vi "Lab Suma total de los valores de un arreglo.vi"() -> ()   [LabVIEW 2018]
uses:
  <vilib>/Analysis/baseanly.llb/Mean (DBL).vi
  <vilib>/Analysis/NI_AALBase.lvlib
panel:
  out "Numeric 2":dbl
  out "promedio":dbl format="%0.2f"
  out "Minimo Indexado":i32
  out "Maximo Indexado":i32
  out "Minimo":dbl
  out "Maximo":dbl
  out "Array":dbl[](array[numeric])
  out "Numeric":dbl
  in  "Knob":dbl(knob) scale=0.0..10.0
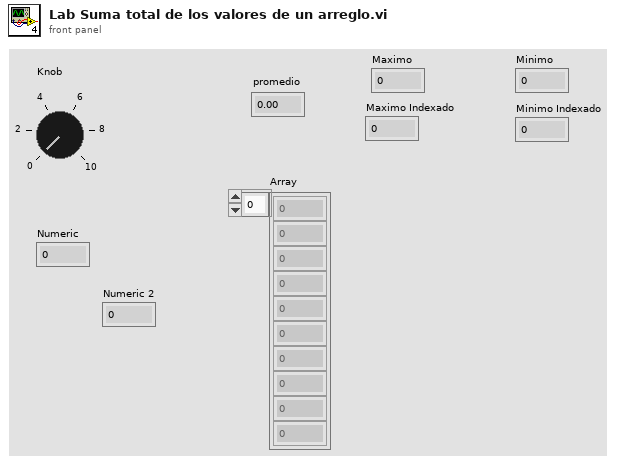
[diagram p1: front panel]
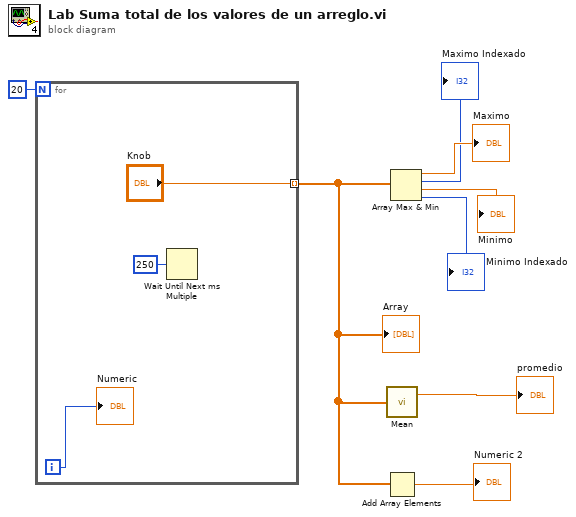
[diagram p0: block diagram]
diagram:
  n1 = for {
    N: 20 -> [_]
    tunnel: ["Knob"] -> w2 mode=indexing
    i -> [w9]
    n2 = Wait Until Next ms Multiple(millisecond multiple=u32 250) -> ()  [unwired: 1 out]
    "Numeric" <- w9
  }
  "Array" <- w2
  n3 = call-poly <vilib>:"Mean.vi"("X"=w2) -> ("mean"=→"promedio":dbl)  [unwired: 1 out]
  n4 = Add Array Elements(numeric array=w2) -> (sum=→"Numeric 2":dbl)
  n5 = Array Max & Min(array=w2) -> (max value=→"Maximo":dbl, max index (indices)=→"Maximo Indexado":i32, min value=→"Minimo":dbl, min index (indices)=→"Minimo Indexado":i32)
